vi "variant0.vi"() -> ()   [LabVIEW 2016]
panel:
  in  "Stop Button":bool
  out "variant":variant
  in  "String":string
  in  "Boolean":bool
  in  "Numeric Control":dbl
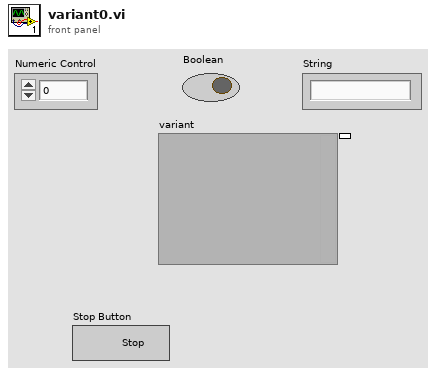
[diagram p1: front panel]
types:
  T1 = enum16{"Read", "Write", "ReadWrite", "BufferedRead", "BufferedReadWrite"}
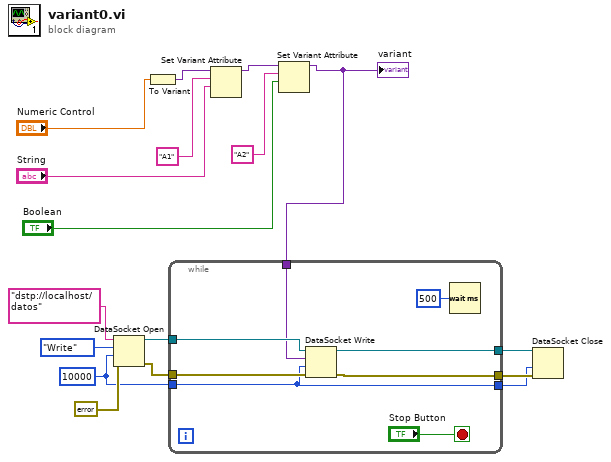
[diagram p0: block diagram]
diagram:
  w7 = 10000 ("ms timeout (10000)")
  n1 = DataSocket Open(8:errorcluster {"status"=FALSE, "code"=0, "source"=""} ("error in (no error)"), 9:w7, 10:T1."Write" ("mode"), 11:"dstp://localhost/datos" ("connection in")) -> (0:w5:errorcluster, 3:w6:refnum<k13>)
  n2 = To Variant(anything="Numeric Control") -> (Variant=w17:variant)
  n3 = Set Variant Attribute(Variant=w17, name="A1", value="String") -> (Variant out=w13:variant)  [unwired: 1 in, 2 out]
  n4 = Set Variant Attribute(Variant=w13, name="A2", value="Boolean") -> (Variant out=w1:variant)  [unwired: 1 in, 2 out]
  "variant" <- w1
  n5 = while {
    tunnel: w7 -> [w19]
    tunnel: w6 -> [w23]
    tunnel: w5 -> [w22]
    tunnel: [w21] -> w4
    tunnel: [w20] -> w3
    tunnel: [w19] -> w2
    tunnel: w1 -> [w18]
    stop <- "Stop Button" stop-if-true
    n6 = DataSocket Write(8:w22, 9:w19, 10:w18, 11:w23) -> (0:w21:errorcluster, 3:w20:refnum<k13>)  [unwired: 1 out]
    n7 = Wait (ms)(milliseconds to wait=u32 500) -> ()  [unwired: 1 out]
  }
  n8 = DataSocket Close(8:w4, 9:w2, 11:w3) -> ()  [unwired: 2 out]
